vi "Configure Sequence File View Manager.vi"(8 "error in (no error)":errorcluster, 11 "TS UI Data in":T1) -> (0 "error out":errorcluster, 3 "TS UI Data out":T1)   [LabVIEW 2015]
uses:
  Type defs/TS UI Data.ctl
  Type defs/Nest cluster.ctl
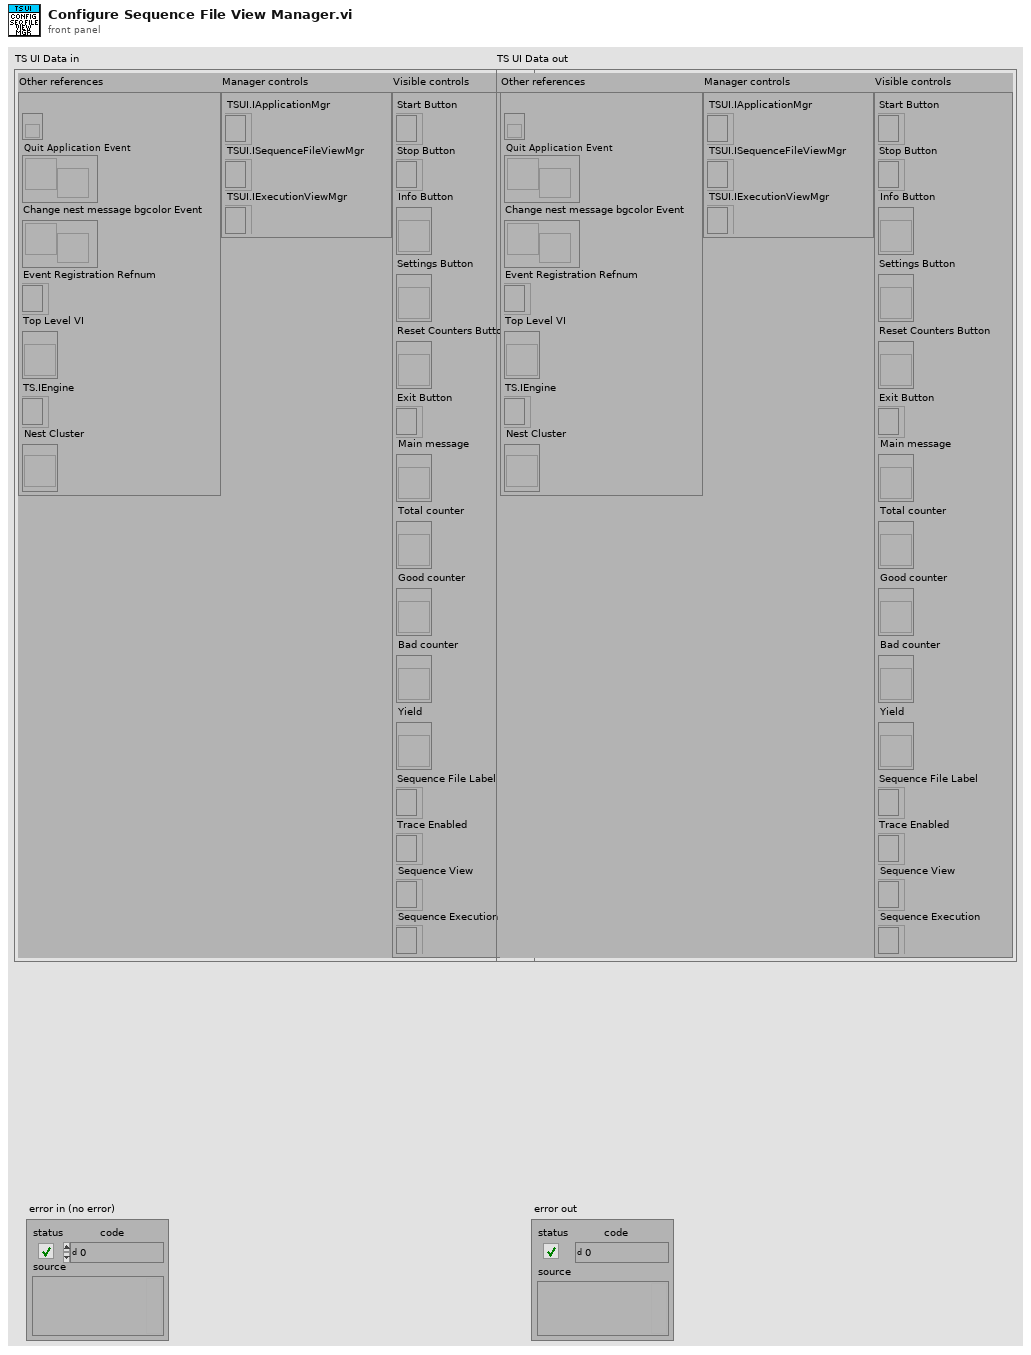
[diagram p1: front panel]
types:
  T1 = typedef "TS UI Data.ctl" = cluster{"Other references":cluster{"event callback refnum":refnum<k27>, "Quit Application Event":refnum<user-event>, "Change nest message bgcolor Event":refnum<user-event>, "event registration refnum":refnum<event-registration>, "Top Level VI":refnum<vi>, "TS.IEngine":refnum<k7>, "Nest Cluster":refnum<vi>}, "Manager controls":cluster{"TSUI.IApplicationMgr":refnum<k7>, "TSUI.ISequenceFileViewMgr":refnum<k7>, "TSUI.IExecutionViewMgr":refnum<k7>}, "Visible controls":cluster{"Start Button":refnum<k7>, "Stop Button":refnum<k7>, "Info Button":refnum<vi>, "Settings Button":refnum<vi>, "Reset Counters Button":refnum<vi>, "Exit Button":refnum<k7>, "Main message":refnum<vi>, "Total counter":refnum<vi>, "Good counter":refnum<vi>, "Bad counter":refnum<vi>, "Yield":refnum<vi>, "Sequence File Label":refnum<k7>, "Trace Enabled":refnum<k7>, "Sequence View":refnum<k7>, "Sequence Execution":refnum<k7>}}
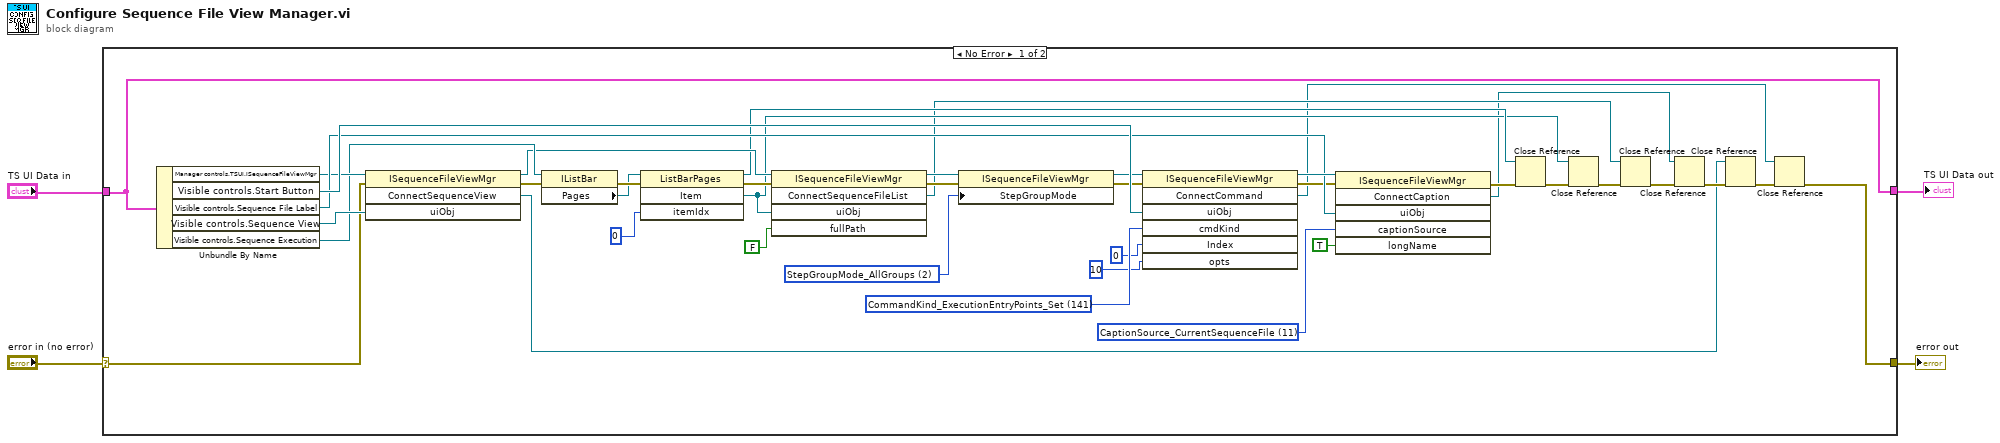
[diagram p0: block diagram]
diagram:
  n1 = case shown="No Error" "error in (no error)" {
    selector: "error in (no error)" -> [w31 w45]
    tunnel: "TS UI Data in" -> [w40 w44]
    tunnel: [w40 w44] -> w2
    tunnel: [w6 w45] -> w1
    frame No Error {
      w18 = 2 items=["StepGroupMode_OneGroup"=1, "StepGroupMode_AllGroups"=2] ("StepGroupMode")
      w35 = 11 items=["CaptionSource_NotASource", "CaptionSource_MacroExpression", "CaptionSource_UUTSerialNumber", "CaptionSource_UUTStatus", "CaptionSource_BatchSerialNumber", "CaptionSource_BatchStatus", "CaptionSource_BatchState", "CaptionSource_ModelState", "CaptionSource_UserName", "CaptionSource_ProgressText", "CaptionSource_ProgressPercent", "CaptionSource_CurrentSequenceFile", "CaptionSource_CurrentSequenceFileComment", "CaptionSource_CurrentSequence", "CaptionSource_CurrentSequenceComment", "CaptionSource_CurrentStepGroup", "CaptionSource_CurrentStep", "CaptionSource_CurrentStepComment", "CaptionSource_CurrentStepIndex_ZeroBased", "CaptionSource_CurrentTestIndex_OneBased", "CaptionSource_SelectedSteps_ZeroBased", "CaptionSource_SelectedTests_OneBased", "CaptionSource_NumberOfSteps", "CaptionSource_NumberOfTests", "CaptionSource_CurrentExecution", "CaptionSource_CurrentThread", "CaptionSource_CurrentCallStackEntry", "CaptionSource_CurrentProcessModelFile", "CaptionSource_ReportLocation", "CaptionSource_TestSocketIndex", "CaptionSource_Time", "CaptionSource_Date", "CaptionSource_CurrentSequenceFile_WithoutFileState", "CaptionSource_CurrentSequenceFile_FileStateOnly"] ("captionSource")
      w42 = 141 items=["CommandKind_NotACommand"=0, "CommandKind_Container"=1, "CommandKind_Separator"=2, "CommandKind_Custom"=3, "CommandKind_OpenSequenceFile"=20, "CommandKind_Close"=21, "CommandKind_CloseAll"=22, "CommandKind_CloseCompletedExecutions"=23, "CommandKind_OpenWorkspaceBrowser"=24, "CommandKind_Login"=25, "CommandKind_Logout"=26, "CommandKind_LoginLogout"=27, "CommandKind_UnloadAllModules"=28, "CommandKind_MRUFile"=29, "CommandKind_Exit"=30, "CommandKind_Restart"=40, "CommandKind_RunEntryPoint"=41, "CommandKind_RunEntryPointOnSelectedSteps"=42, "CommandKind_LoopEntryPointOnSelectedSteps"=43, "CommandKind_RunCurrentSequence"=44, "CommandKind_RunSpecificSequence"=45, "CommandKind_RunSelectedSteps"=46, "CommandKind_RunSelectedStepsUsingEntryPointsSubmenu"=47, "CommandKind_LoopOnSelectedSteps"=48, "CommandKind_LoopOnSelectedStepsUsingEntryPointsSubmenu"=49, "CommandKind_BreakOnFirstStep"=50, "CommandKind_BreakOnStepFailure"=51, "CommandKind_BreakOnSequenceFailure"=52, "CommandKind_TracingEnabled"=53, "CommandKind_ToggleBreakpoint"=60, "CommandKind_SetRunModeSubmenu"=61, "CommandKind_RunModeForcePass"=62, "CommandKind_RunModeForceFail"=63, "CommandKind_RunModeSkip"=64, "CommandKind_RunModeNormal"=65, "CommandKind_Resume"=66, "CommandKind_StepInto"=67, "CommandKind_StepOver"=68, "CommandKind_StepOut"=69, "CommandKind_SetNextStep"=70, "CommandKind_Break"=71, "CommandKind_BreakResume"=72, "CommandKind_Terminate"=73, "CommandKind_TerminateRestart"=74, "CommandKind_Abort"=75, "CommandKind_BreakAll"=76, "CommandKind_TerminateAll"=77, "CommandKind_AbortAll"=78, "CommandKind_ResumeAll"=79, "CommandKind_DisplayBreakpointsAndWatchExpressions"=80, "CommandKind_DisplayBreakpointSettings"=81, "CommandKind_BreakpointSubmenu"=85, "CommandKind_ConfigureAdapters"=90, "CommandKind_ConfigureStationOptions"=91, "CommandKind_ConfigureSearchDirectories"=92, "CommandKind_ConfigureExternalViewers"=93, "CommandKind_ToolItem"=100, "CommandKind_CustomizeTools"=101, "CommandKind_ExecutionEntryPointInsertionMarker"=110, "CommandKind_ExecutionEntryPointDefaultMenuInsertionMarker"=111, "CommandKind_ConfigurationEntryPointInsertionMarker"=112, "CommandKind_ConfigurationEntryPointDefaultMenuInsertionMarker"=113, "CommandKind_SequenceViewConfiguration"=116, "CommandKind_SequenceViewConfigurationsSubmenu"=118, "CommandKind_DefaultFileMenu_Set"=120, "CommandKind_DefaultExecuteMenu_Set"=121, "CommandKind_DefaultDebugMenu_Set"=123, "CommandKind_DefaultConfigureMenu_Set"=124, "CommandKind_DefaultToolsMenu_Set"=125, "CommandKind_DefaultSequenceViewContextMenu_Set"=126, "CommandKind_DefaultListBarContextMenu_Set"=127, "CommandKind_DefaultEditMenu_Set"=128, "CommandKind_DefaultSequenceListContextMenu_Set"=129, "CommandKind_SequenceViewConfigurations_Set"=139, "CommandKind_MRUFiles_Set"=140, "CommandKind_ExecutionEntryPoints_Set"=141, "CommandKind_RunSequences_Set"=142, "CommandKind_RunSelectedStepsUsingEntryPoints_Set"=143, "CommandKind_LoopOnSelectedStepsUsingEntryPoints_Set"=144, "CommandKind_ConfigurationEntryPoints_Set"=145, "CommandKind_Tools_Set"=146, "CommandKind_OpenSequenceFiles"=147, "CommandKind_LockUnlock"=148, "CommandKind_ConfigureSequenceViews"=149, "CommandKind_Edit_Undo"=200, "CommandKind_Edit_Redo"=201, "CommandKind_Edit_Rename"=202, "CommandKind_Edit_Cut"=203, "CommandKind_Edit_Copy"=204, "CommandKind_Edit_Paste"=205, "CommandKind_Edit_Delete"=206, "CommandKind_Edit_InsertStep"=207, "CommandKind_Edit_Save"=208, "CommandKind_Edit_SaveAs"=209, "CommandKind_Edit_SaveAll"=210, "CommandKind_Edit_NewSequenceFile"=211, "CommandKind_Edit_StepProperties"=212, "CommandKind_Edit_SequenceProperties"=213, "CommandKind_Edit_SequenceFileProperties"=214, "CommandKind_Edit_SpecifyModule"=215, "CommandKind_Edit_EditCode"=216, "CommandKind_Edit_EditStep"=217, "CommandKind_Edit_Preconditions"=218, "CommandKind_SelectAll"=219, "CommandKind_Edit_SelectDefaultAdapter"=220, "CommandKind_Edit_InsertSequence"=221, "CommandKind_Edit_SequenceFileCallbacks"=222, "CommandKind_Edit_EditPaths"=223, "CommandKind_Edit_EncapsulateSelectedSteps"=224, "CommandKind_Edit_InsertStepsSubmenu"=300, "CommandKind_Edit_EditStepsSubmenu"=301, "CommandKind_Edit_SelectDefaultAdaptersSubmenu"=302, "CommandKind_Edit_EncapsulateSelectedStepsSubmenu"=303, "CommandKind_Edit_InsertSteps_Set"=340, "CommandKind_Edit_EditSteps_Set"=341, "CommandKind_Edit_SelectDefaultAdapters_Set"=342, "CommandKind_Edit_EncapsulateSelectedSteps_Set"=343, "CommandKind_ShowInList"=400, "CommandKind_ShowInVariables"=401, "CommandKind_ShowTestStandHelp"=420, "CommandKind_ShowGuideToDocumentation"=421, "CommandKind_ShowHelpTopic"=422, "CommandKind_ShowTestStandWebResources"=423, "CommandKind_ShowTestStandDiscussionForum"=424, "CommandKind_ShowPatents"=425, "CommandKind_DefaultHelpMenu_Set"=440, "CommandKind_Edit_Attributes"=450, "CommandKind_Edit_AdvancedSequenceListSubmenu"=451, "CommandKind_ShowUpdateService"=452, "CommandKind_ShowExamples"=453, "CommandKind_ShowGettingStarted"=454] ("cmdKind")
      n2 = Unbundle By Name(w40) -> ("Manager controls.TSUI.ISequenceFileViewMgr"=w32:refnum<k7>, "Visible controls.Start Button"=w43:refnum<k7>, "Visible controls.Sequence File Label"=w38:refnum<k7>, "Visible controls.Sequence View"=w33:refnum<k7>, "Visible controls.Sequence Execution"=w29:refnum<k7>)
      n3 = invoke class="ISequenceFileViewMgr" method="ConnectSequenceView"(reference=w32, error in=w31, "uiObj"=w33) -> (reference out=w24:refnum<k7>, error out=w30:errorcluster, "ConnectSequenceView"=w8:refnum<k7>)  [unwired: 1 in, 1 out]
      n4 = property class="IListBar"(reference=w29, error in=w30) -> (error out=w28:errorcluster, "Pages"=w27:refnum<k7>)  [unwired: 1 out]
      n5 = invoke class="ListBarPages" method="Item"(reference=w27, error in=w28, "itemIdx"=0) -> (reference out=w16:refnum<k7>, error out=w25:errorcluster, "Item"=w14:refnum<k7>)  [unwired: 1 in, 1 out]
      n6 = invoke class="ISequenceFileViewMgr" method="ConnectSequenceFileList"(reference=w24, error in=w25, "uiObj"=w14, "fullPath"=FALSE) -> (reference out=w20:refnum<k7>, error out=w22:errorcluster, "ConnectSequenceFileList"=w12:refnum<k7>)  [unwired: 1 in, 2 out]
      n7 = property class="ISequenceFileViewMgr"(reference=w20, error in=w22, "StepGroupMode"=w18) -> (reference out=w19:refnum<k7>, error out=w21:errorcluster)
      n8 = invoke class="ISequenceFileViewMgr" method="ConnectCommand"(reference=w19, error in=w21, "uiObj"=w43, "cmdKind"=w42, "Index"=0, "opts"=10) -> (reference out=w39:refnum<k7>, error out=w37:errorcluster, "ConnectCommand"=w5:refnum<k7>)  [unwired: 1 in, 4 out]
      n9 = invoke class="ISequenceFileViewMgr" method="ConnectCaption"(reference=w39, error in=w37, "uiObj"=w38, "captionSource"=w35, "longName"=TRUE) -> (error out=w17:errorcluster, "ConnectCaption"=w10:refnum<k7>)  [unwired: 1 in, 4 out]
      n10 = Close Reference(reference=w16, error in (no error)=w17) -> (error out=w15:errorcluster)
      n11 = Close Reference(reference=w14, error in (no error)=w15) -> (error out=w13:errorcluster)
      n12 = Close Reference(reference=w12, error in (no error)=w13) -> (error out=w11:errorcluster)
      n13 = Close Reference(reference=w10, error in (no error)=w11) -> (error out=w9:errorcluster)
      n14 = Close Reference(reference=w8, error in (no error)=w9) -> (error out=w7:errorcluster)
      n15 = Close Reference(reference=w5, error in (no error)=w7) -> (error out=w6:errorcluster)
    }
    frame Error {
    }
  }
  "TS UI Data out" <- w2
  "error out" <- w1
